vi "GetParam.vi"(8 "error in (no error)":errorcluster caption="entrée d'erreur (pas d'erreur)", 11 "Euclidean_distances.lvclass":refnum<class "Euclidean_distances.lvclass">) -> (0 "error out":errorcluster caption="sortie d'erreur", 2 "euclidean_distances":T1, 3 "Euclidean_distances.lvclass":refnum<class "Euclidean_distances.lvclass">)   [LabVIEW 2020, in "Euclidean_distances.lvclass"]
doc: "Get Parameters"
uses:
  Euclidean_distances.lvclass
  Euclidean_distances.lvclass/Euclidean_distances.ctl
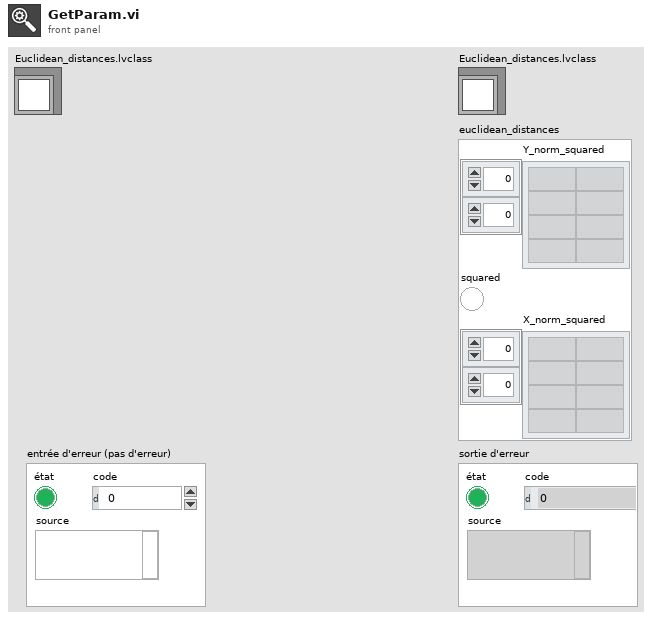
[diagram p1: front panel]
types:
  T1 = cluster{"Y_norm_squared":string[][], "squared":bool, "X_norm_squared":string[][]}
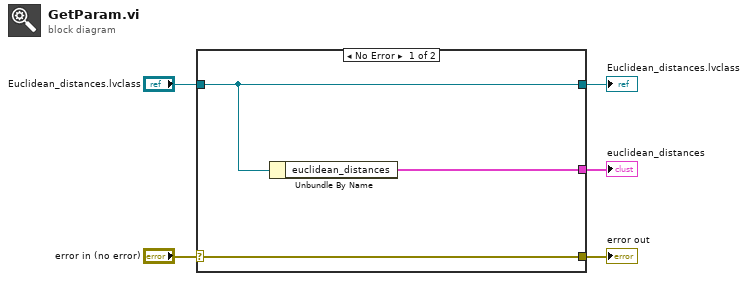
[diagram p0: block diagram]
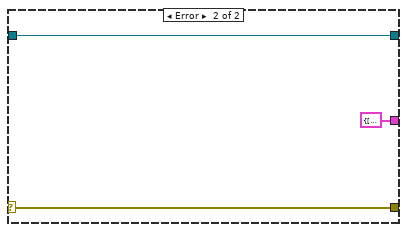
[diagram p2: hidden frame]
diagram:
  n1 = case shown="No Error" "error in (no error)" {
    selector: "error in (no error)" -> [w8 w10]
    tunnel: [w8 w10] -> w4
    tunnel: [w7 w11] -> w2
    tunnel: "Euclidean_distances.lvclass" -> [w7 w11]
    tunnel: [w6 T1 {"Y_norm_squared"=[], "squared"=FALSE, "X_norm_squared"=[]} ("euclidean_distances")] -> w1
    frame No Error {
      n2 = Unbundle By Name(w7) -> ("euclidean_distances"=w6:T1)
    }
    frame Error {
    }
  }
  "error out" <- w4
  "Euclidean_distances.lvclass" <- w2
  "euclidean_distances" <- w1
